vi "TLTSP_Initialize.vi"(8 "error in (no error)":errorcluster, 9 "Query ID?":bool, 10 "Reset":bool, 11 "VISA In":refnum<visa-resource-name>) -> (0 "error out":errorcluster, 2 "read buffer":string, 3 "VISA Out":refnum<visa-resource-name>)   [LabVIEW 2017]
panel:
  out "Status Byte":i32
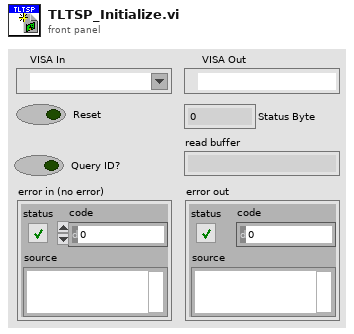
[diagram p1: front panel]
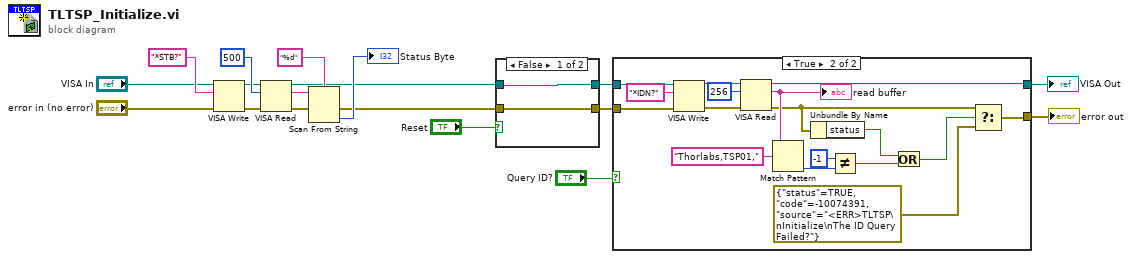
[diagram p0: block diagram]
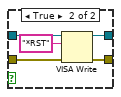
[diagram p3: hidden frame]
diagram:
  n1 = VISA Write(VISA resource name="VISA In", write buffer="*STB?", error in (no error)="error in (no error)") -> (VISA resource name out=w14:refnum<visa-resource-name>, error out=w13:errorcluster)  [unwired: 1 out]
  n2 = VISA Read(VISA resource name=w14, byte count=u32 500, error in (no error)=w13) -> (VISA resource name out=w4:refnum<visa-resource-name>, read buffer=w9:string, error out=w3:errorcluster)  [unwired: 1 out]
  n3 = Scan From String(format string="%d", input string=w9) -> (output 1=→"Status Byte":i32)  [unwired: 3 in, 3 out]
  n4 = case shown="False" "Reset" {
    tunnel: w4 -> [w18 w24]
    tunnel: w3 -> [w19 w23]
    tunnel: [w19 w21] -> w17
    tunnel: [w18 w20] -> w16
    frame False {
    }
    frame True {
      n5 = VISA Write(VISA resource name=w24, write buffer="*RST", error in (no error)=w23) -> (VISA resource name out=w20:refnum<visa-resource-name>, error out=w21:errorcluster)  [unwired: 1 out]
    }
  }
  n6 = case shown="True" "Query ID?" {
    tunnel: w17 -> [w25 w43]
    tunnel: w16 -> [w26 w42]
    tunnel: [w26 w40] -> w8
    tunnel: [w25 w29] -> w7
    frame False {
    }
    frame True {
      n7 = VISA Write(VISA resource name=w42, write buffer="*IDN?", error in (no error)=w43) -> (VISA resource name out=w38:refnum<visa-resource-name>, error out=w39:errorcluster)  [unwired: 1 out]
      n8 = VISA Read(VISA resource name=w38, byte count=u32 256, error in (no error)=w39) -> (VISA resource name out=w40:refnum<visa-resource-name>, read buffer=w36:string, error out=w27:errorcluster)  [unwired: 1 out]
      "read buffer" <- w36
      n9 = Match Pattern(string=w36, regular expression="Thorlabs,TSP01,") -> (offset past match=w34:i32)  [unwired: 1 in, 3 out]
      n10 = Unbundle By Name(w27) -> ("status"=w30:bool)
      n11 = Not Equal?(x=-1, y=w34) -> (x != y?=w32:bool)
      n12 = Or(x=w30, y=w32) -> (x .or. y?=w31:bool)
      n13 = Select(t=w27, s=w31, f=errorcluster {"status"=TRUE, "code"=-10074391, "source"="<ERR>TLTSP\nInitialize\nThe ID Query Failed?"}) -> (s? t:f=w29:errorcluster)
    }
  }
  "error out" <- w7
  "VISA Out" <- w8
